vi "CirculateBall.vi"(0 "CirculateSkill in":refnum<class "CirculateSkill.lvclass">, 5 "Robot":refnum<class "Robot.lvclass">, 7 "BallRef":refnum<class "Ball.lvclass">, 9 "Clockwise?":bool, 11 "error in (no error)":errorcluster, 12 "Skills.CirculateBall":T1={"rotationAngle"=86.0, "velocityFactor"=1.7, "OrientationFactor"=-1.0} {"rotationAngle" format="%#_13g"}) -> (4 "CirculateSkill out":refnum<class "CirculateSkill.lvclass">, 6 "Robot out":refnum<class "Robot.lvclass">, 15 "error out":errorcluster)   [LabVIEW 2023, in "CirculateSkill.lvclass"]
uses:
  CirculateSkill.lvclass
  Ball_class/Ball.lvclass
  C:/Users/ebert/Documents/codes/SSL/repo/SSL_AI/Object_class/Object.lvclass
  Robot_class/Robot.lvclass
  CIrculateSkillParameters.ctl
  Object_class/Object.lvclass/Object.ctl
  Object_class/Read position(x,y).vi
  CirculateSkill.lvclass/CirculateSkill.ctl
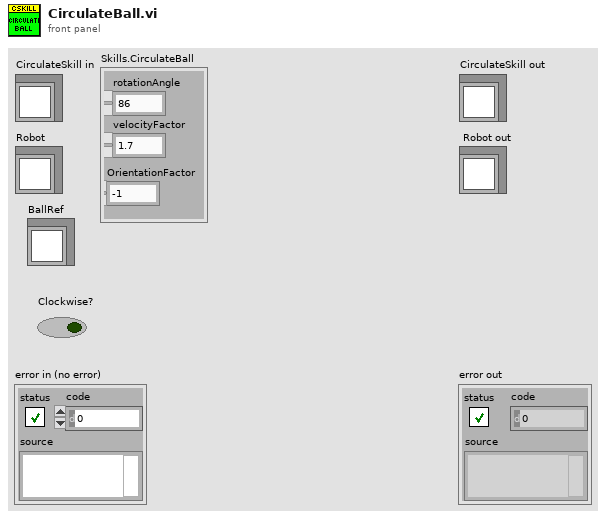
[diagram p1: front panel]
types:
  T1 = typedef "CIrculateSkillParameters.ctl" = cluster{"rotationAngle":dbl, "velocityFactor":dbl, "OrientationFactor":dbl}
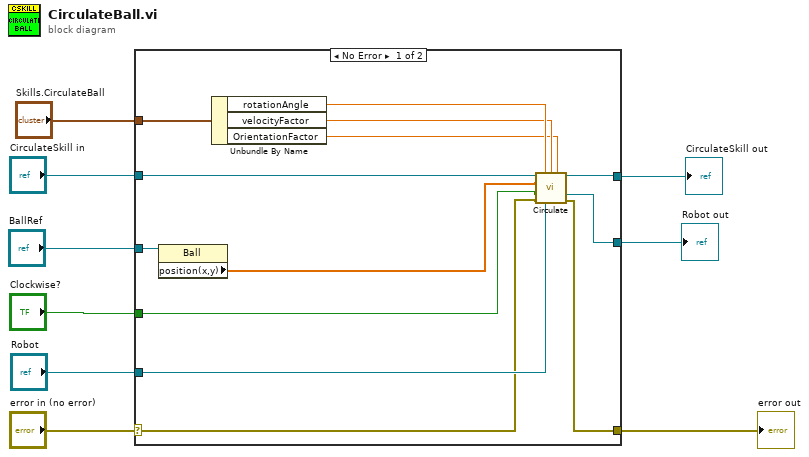
[diagram p0: block diagram]
diagram:
  n1 = case shown="No Error" "error in (no error)" {
    selector: "error in (no error)" -> [w17 w25]
    tunnel: [w14 w25] -> w8
    tunnel: [w16 w24] -> w6
    tunnel: "CirculateSkill in" -> [w21 w24]
    tunnel: "BallRef" -> [w22 _]
    tunnel: "Clockwise?" -> [w19 _]
    tunnel: "Robot" -> [w18 w23]
    tunnel: [w15 w23] -> w2
    tunnel: "Skills.CirculateBall" -> [w10 _]
    frame No Error {
      n2 = property class="Ball"(reference=w22) -> ("position(x,y)"=w20:dbl[])  [unwired: 1 in, 2 out]
      n3 = Unbundle By Name(w10) -> ("rotationAngle"=w13:dbl, "velocityFactor"=w12:dbl, "OrientationFactor"=w11:dbl)
      n4 = call-dynamic "Circulate.vi"("CirculateSkill in"=w21, "rotationAngle"=w13, "velocityFactor"=w12, "OrientationFactor"=w11, "Target"=w20, "Clockwise?"=w19, "error in (no error)"=w17, "Robot"=w18) -> ("CirculateSkill out"=w16:refnum<class "CirculateSkill.lvclass">, "Robot out"=w15:refnum<class "Robot.lvclass">, "error out"=w14:errorcluster)  [unwired: 5 in]
    }
    frame Error {
    }
  }
  "error out" <- w8
  "CirculateSkill out" <- w6
  "Robot out" <- w2
